vi "Read Process.vi"(8 "error in (no error)":errorcluster, 11 "Process Test in":refnum<class "Process Test.lvclass">) -> (0 "error out":errorcluster, 2 "Process.lvclass":refnum<class "Process.lvclass">, 3 "Process Test out":refnum<class "Process Test.lvclass">)   [LabVIEW 2020, in "Process Test.lvclass"]
uses:
  Process Test.lvclass
  Framework/Process/Process.lvclass
  C:/Users/anton/Documents/GitHub/Triarc/source/Framework Test/Base Class Test/Base Class Test.lvclass
  Base Class Test/Base Class Test.lvclass/Base Class Test.ctl
  Framework/Base/Base.lvclass
  Base Class Test/Base Class Test.lvclass
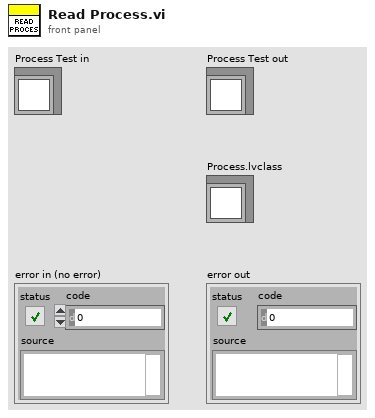
[diagram p1: front panel]
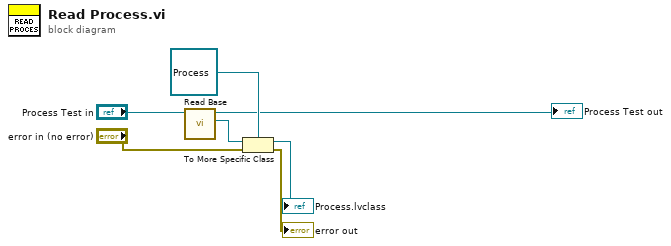
[diagram p0: block diagram]
diagram:
  n1 = call "Read Base.vi"("Base Class Test In"="Process Test in") -> ("Base.lvclass"=w4:refnum<class "Base.lvclass">, "Base Class Test Out"=→"Process Test out":refnum<class "Process Test.lvclass">)  [unwired: 8 in, 1 out]
  n2 = To More Specific Class(target class=refnum<class "Process.lvclass"> refnum ("Process.lvclass"), reference=w4, error in="error in (no error)") -> (specific class reference=→"Process.lvclass":refnum<class "Process.lvclass">, error out=→"error out":errorcluster)
